vi "AutoFileCreatorMain.vi"() -> ()   [LabVIEW 2017]
uses:
  <vilib>/Utility/inputDevices.llb/mouseAcquire.vi
  <vilib>/xml/NI_XML.lvlib
  <resource>/objmgr/DOMUserDefRef.rc
panel:
  out "CopiedData":string
  in  "LocalFileNames":string[](array[string])=["1A.txt", "1B.txt", "1C.txt", "1D.txt", "2A.txt", "2B.txt", "2C.txt", "2D.txt", "3A.txt", "3B.txt", "3C.txt", "3D.txt", "4A.txt", "4B.txt", "4C.txt", "4D.txt"]
  out "standard output":string
  out "standard error":string="NI Linux Real-Time (run mode)\n\nLog in with your NI-Auth credentials.\n\n"
  in  "LocalFiles":i32(listbox)=2
  in  "SaveToLocal":bool
  in  "LoadFromLocal":bool
  in  "ExportToRobot":bool
  out "XML With IDs":string="<Sequential ID=\"1\">\n</Sequential>"
  in  "Commands":i32(listbox)=-1
  out "XML":string="<Sequential>\n</Sequential>"
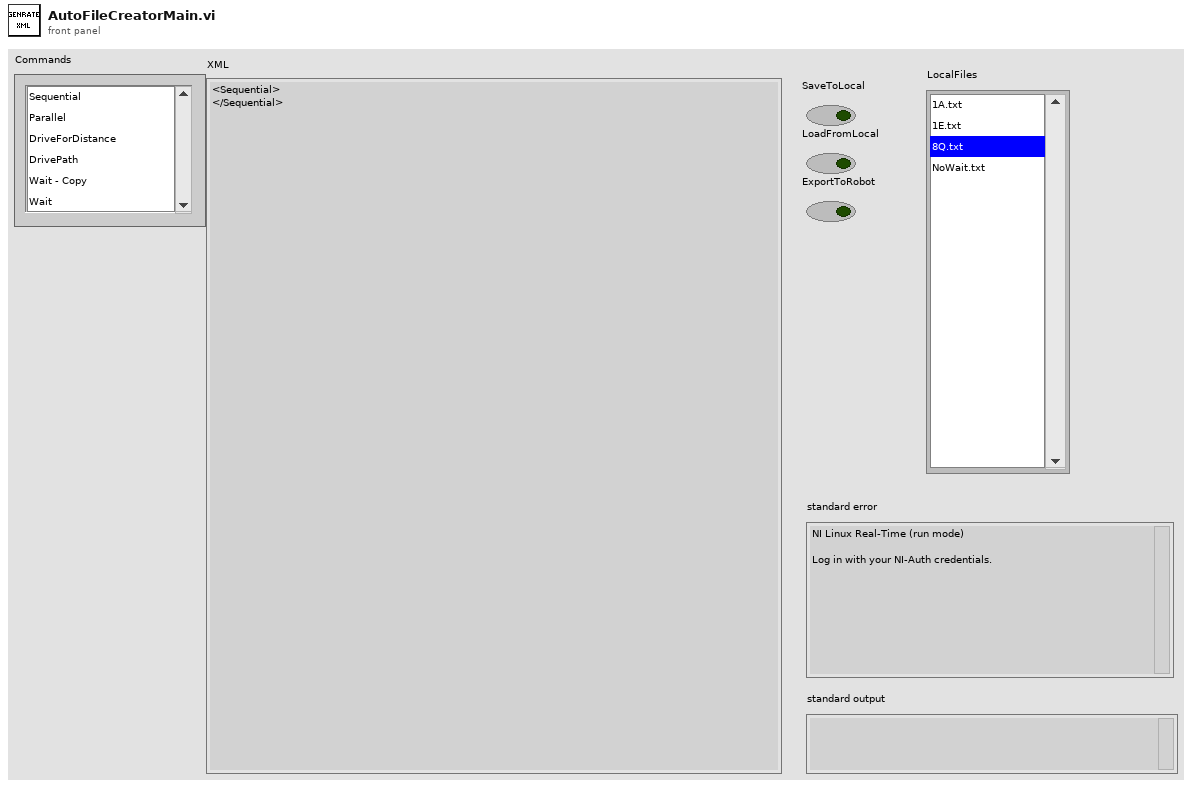
[diagram p1: front panel]
types:
  T1 = cluster{"Horizontal":i32, "Vertical":i32, "Scrolling":i32}
  T2 = typedef "eventvkey.ctl" = enum16{"ASCII", "Enter", "Return", "Shift", "Ctrl", "Alt", "Cmd", "Opt", "Caps", "NumLock", "Clear", "Break", "Up", "Down", "Left", "Right", "Insert", "Delete", "Home", "End", "PageUp", "PageDown", "Escape", "Help", "Pause", "ScrollLock", "F1", "F2", "F3", "F4", "F5", "F6", "F7", "F8", "F9", "F10", "F11", "F12", "F13", "F14", "F15", "F16", "F17", "F18", "F19", "F20", "F21", "F22", "F23", "F24", "Play", "VolumeUp", "VolumeDown", "Mute", "Two Byte Char"}
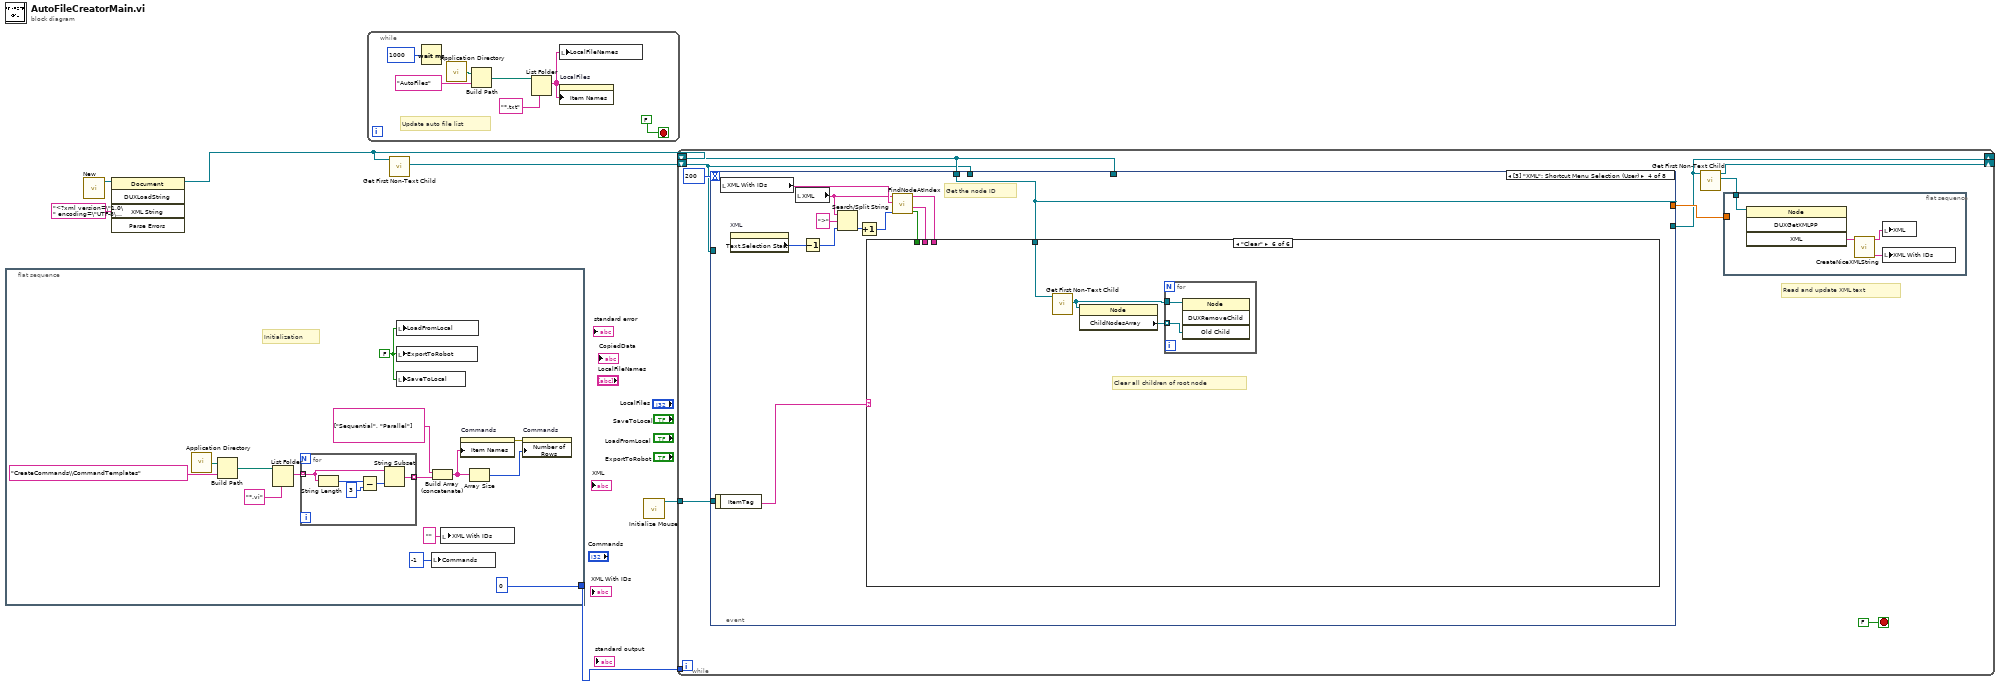
[diagram p0: block diagram]
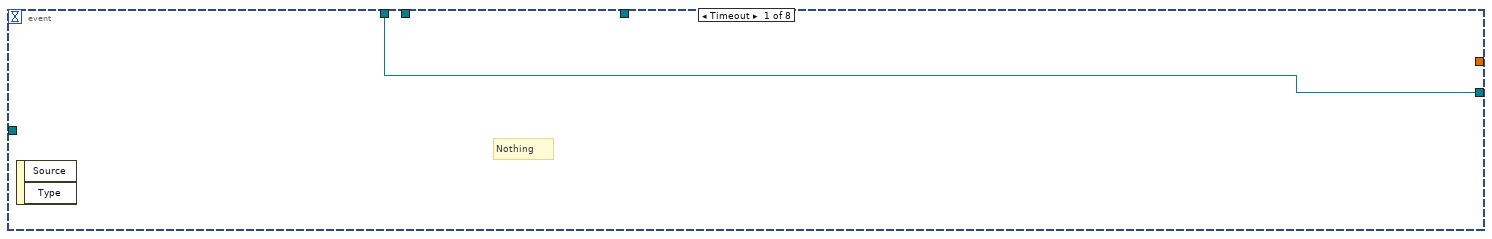
[diagram p2: hidden frame]
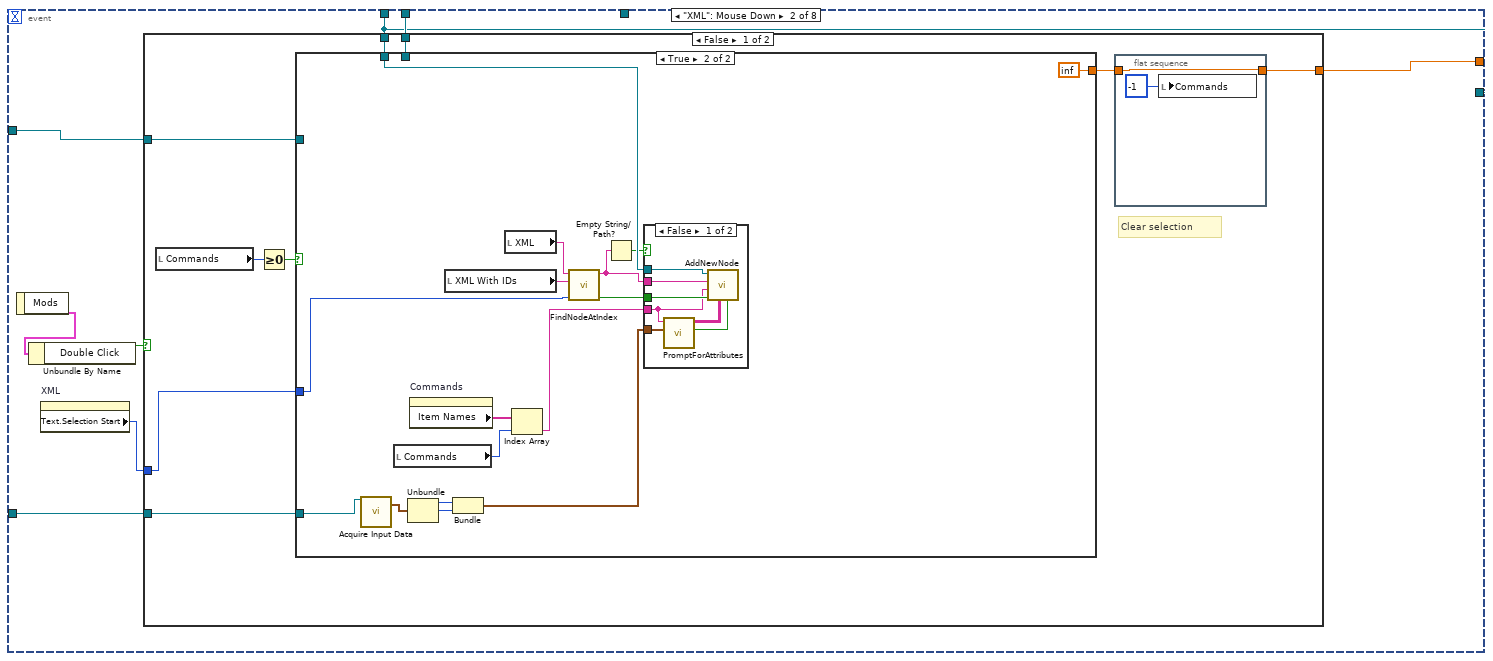
[diagram p3: hidden frame]
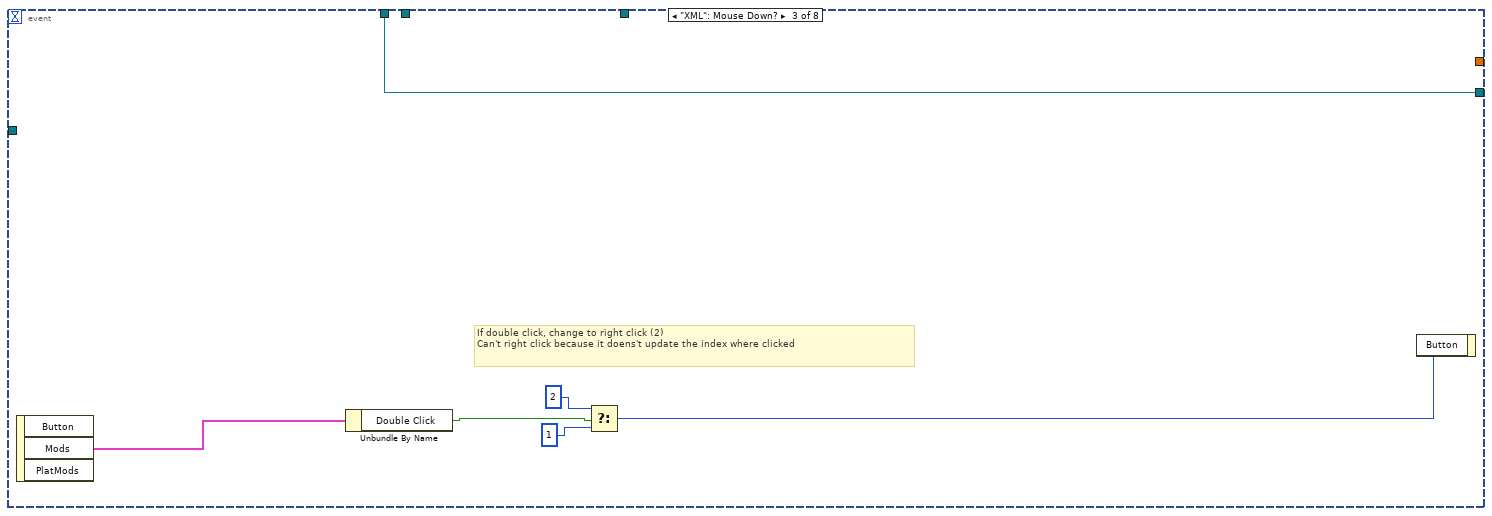
[diagram p7: hidden frame]
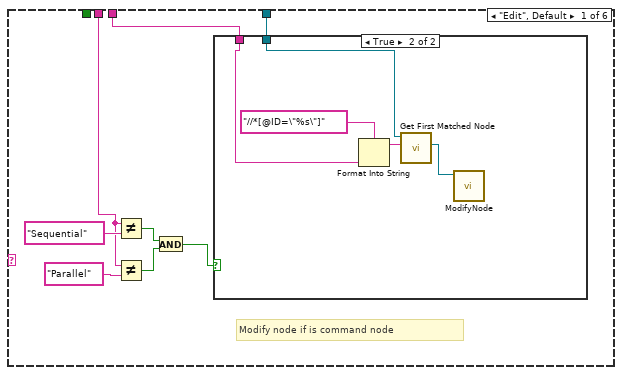
[diagram p8: hidden frame]
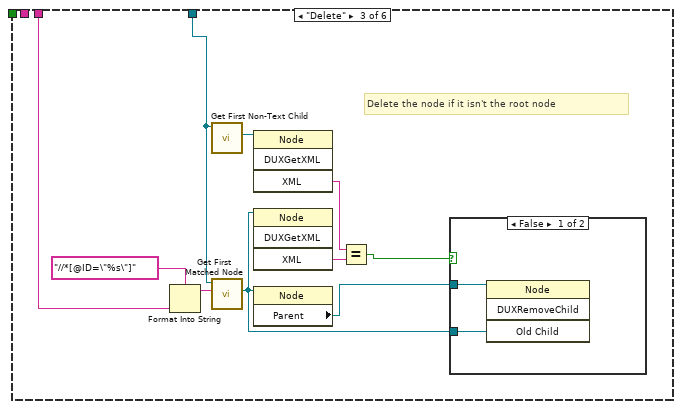
[diagram p11: hidden frame]
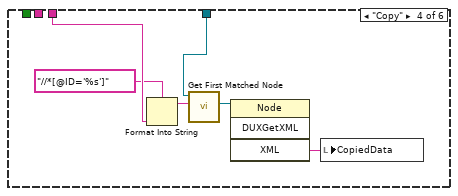
[diagram p13: hidden frame]
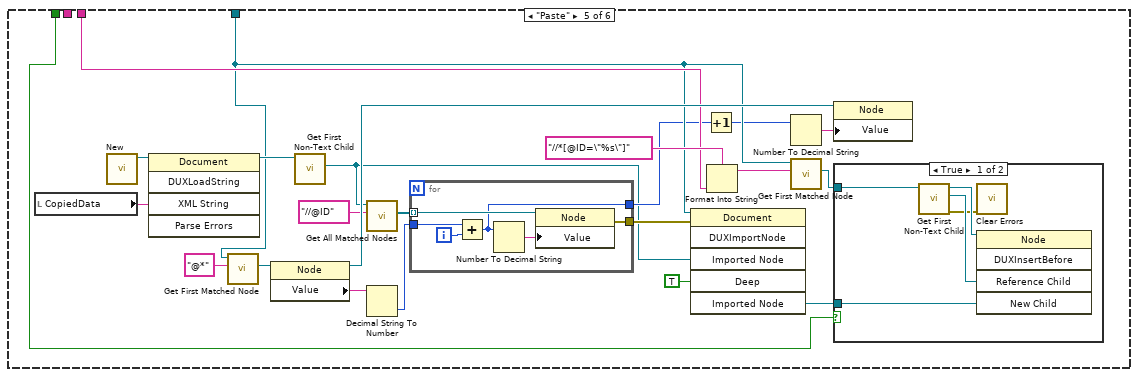
[diagram p14: hidden frame]
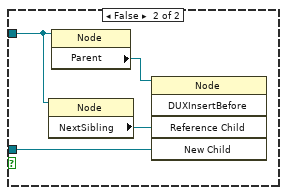
[diagram p15: hidden frame]
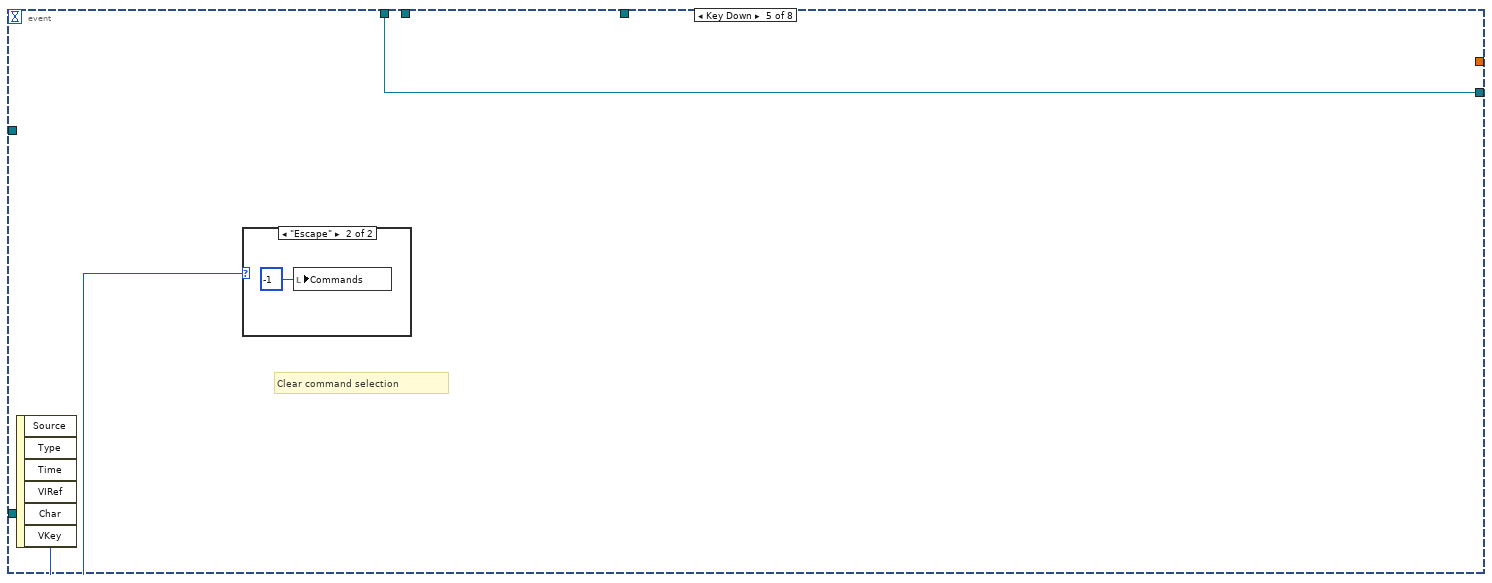
[diagram p16: hidden frame]
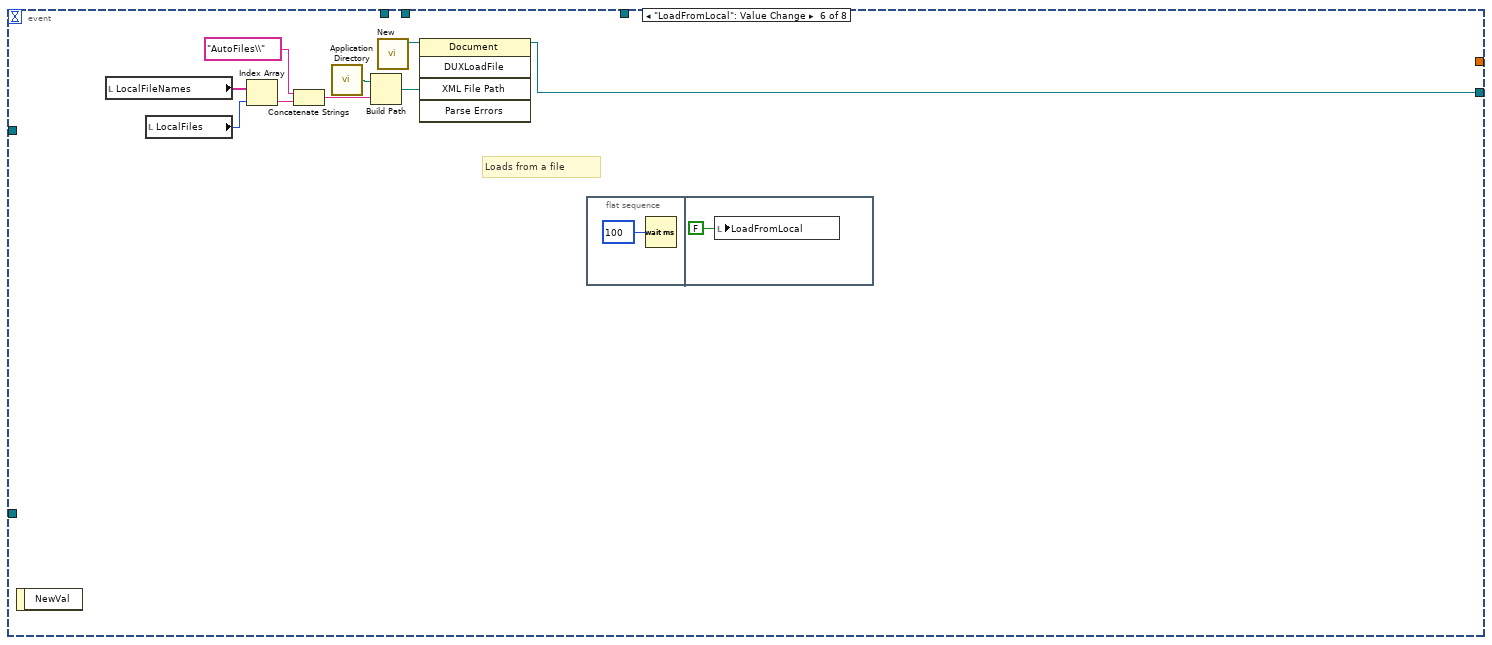
[diagram p18: hidden frame]
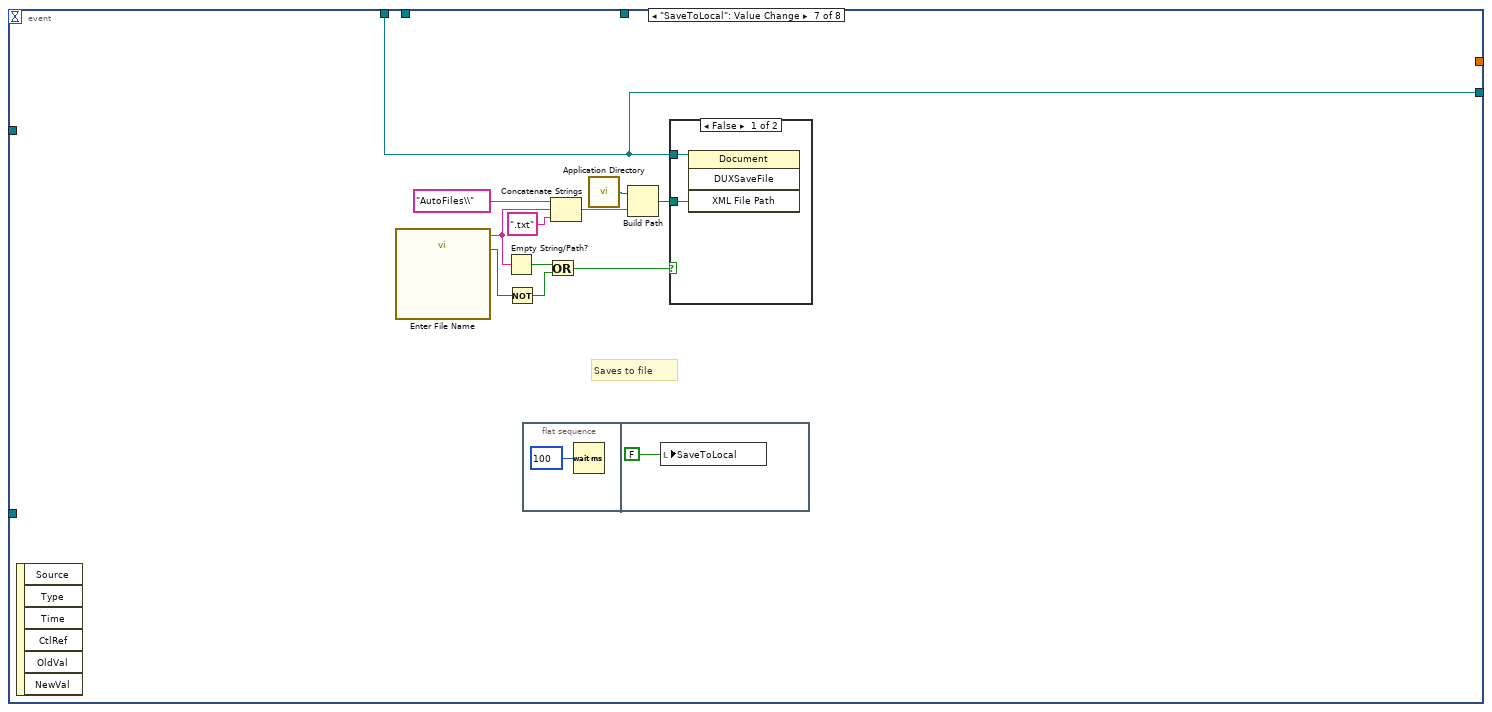
[diagram p19: hidden frame]
diagram:
  n1 = flat-sequence {
    tunnel: [0] -> w6
    frame #0 {
      w7 = FALSE ("SaveToLocal")
      # "Initialization"
      n2 = call <vilib>:"Application Directory.vi"() -> ("Application Directory"=w11:path)
      n3 = Build Path(base path=w11, name or relative path="CreateCommands\\CommandTemplates") -> (appended path=w12:path)
      n4 = List Folder(path=w12, pattern="*.vi") -> (filenames=w13:string[])  [unwired: 2 in, 3 out]
      n5 = for {
        tunnel: w13 -> [w25] mode=indexing
        tunnel: [w21] -> w14 mode=indexing
        n6 = String Length(string=w25) -> (length=w24:i32)
        n7 = Subtract(x=w24, y=3) -> (x-y=w22:i32)
        n8 = String Subset(string=w25, length (rest)=w22) -> (substring=w21:string)  [unwired: 1 in]
      }
      n9 = local write "LoadFromLocal"(w7) -> ()
      n10 = local write "ExportToRobot"(w7) -> ()
      n11 = local write "SaveToLocal"(w7) -> ()
      n12 = local write "Commands"(-1 ("Active Row:Active Row Number")) -> ()
      n13 = Build Array (concatenate)(string[] ["Sequential", "Parallel"], w14) -> (w15:string[])
      n14 = local write "XML With IDs"("" ("XML With IDs")) -> ()
      n15 = property on="Commands" class="LstBox (strict)"("Item Names"=w15) -> (error out=w17:errorcluster)  [unwired: 2 in, 1 out]
      n16 = Array Size(array=w15) -> (size(s)=w16:i32)
      n17 = property on="Commands" class="LstBox (strict)"(error in=w17, "Number of Rows"=w16) -> ()  [unwired: 1 in, 2 out]
    }
  }
  n18 = call <vilib>:"New.vi"() -> ("DOM document out"=w5:refnum<k20>)  [unwired: 8 in, 1 out]
  n19 = invoke class="Document" method="DUXLoadString"(reference=w5, "XML String"="<?xml version=\"1.0\" encoding=\"UTF-8\"?><Sequential ID=\"1\"></Sequential>") -> (reference out=w4:refnum<k20>)  [unwired: 3 in, 4 out]
  n20 = while {
    stop <- FALSE stop-if-true
    # "Update auto file list"
    n21 = Wait (ms)(milliseconds to wait=u32 1000) -> ()  [unwired: 1 out]
    n22 = call <vilib>:"Application Directory.vi"() -> ("Application Directory"=w27:path)
    n23 = Build Path(base path=w27, name or relative path="AutoFiles") -> (appended path=w32:path)
    n24 = List Folder(path=w32, pattern="*.txt") -> (filenames=w26:string[])  [unwired: 2 in, 3 out]
    n25 = local write "LocalFileNames"(w26) -> ()
    n26 = property on="LocalFiles" class="LstBox (strict)"("Item Names"=w26) -> ()  [unwired: 2 in, 2 out]
  }
  n27 = call <vilib>:"Get First Non-Text Child.vi"("node in"=w4) -> ("child node"=w3:refnum<k20>)  [unwired: 7 in, 3 out]
  n28 = call <vilib>:"Initialize Mouse.vi"() -> ("device ID"=w2:refnum<k1>)  [unwired: 10 in, 1 out]
  n29 = while {
    tunnel: w6 -> [_]
    shift-right: [w33] -> _
    shift-left: w4 -> [w37]
    shift-right: [w35] -> _
    shift-left: w3 -> [w36]
    tunnel: w2 -> [w38]
    stop <- FALSE stop-if-true
    # "Read and update XML text"
    n30 = event shown="[3] \"XML\": Shortcut Menu Selection (User)" {
      selector: _ -> [_ _ _ _ _ _ _ _]
      dyn-events: _ -> [_ _ _ _ _ _ _ _]
      timeout: 200 -> [_ _ _ _ _ _ _ _]
      tunnel: w36 -> [_ w54 _ _ _ _ _ _]
      tunnel: w37 -> [w46 w47 w89 w96 w181 _ w195 w210]
      tunnel: w36 -> [_ w53 _ _ _ _ _ _]
      tunnel: [_ w52 _ _ _ _ _ _] -> w39
      tunnel: w38 -> [_ w51 _ _ _ _ _ _]
      tunnel: w37 -> [_ _ _ _ _ _ _ _]
      tunnel: [w46 w47 w89 w96 w181 w184 w195 w210] -> w33
      event Timeout {
        # "Nothing"
        n31 = event-data() -> ()  [unwired: 1 in, 2 out]
      }
      event "XML": Mouse Down {
        n32 = event-data() -> ("Mods"=w50:cluster{"Double Click":bool, "Menu Key":bool})  [unwired: 1 in]
        n33 = Unbundle By Name(w50) -> ("Double Click"=w49:bool)
        n34 = property on="XML" class="Str"() -> ("Text.Selection Start"=w48:u32)  [unwired: 2 in, 2 out]
        n35 = case shown="False" w49 {
          tunnel: w54 -> [w61 _]
          tunnel: w47 -> [w60 _]
          tunnel: w53 -> [w59 _]
          tunnel: [w57 _] -> w52
          tunnel: w51 -> [w56 _]
          tunnel: w48 -> [w55 _]
          frame False {
            # "Clear selection"
            n36 = local read "Commands"() -> (w63:i32)
            n37 = Greater Or Equal To 0?(x=w63) -> (x >= 0?=w62:bool)
            n38 = case shown="True" w62 {
              tunnel: w61 -> [_ _]
              tunnel: w60 -> [_ w72]
              tunnel: w59 -> [_ _]
              tunnel: w55 -> [_ w76]
              tunnel: [_ inf] -> w58
              tunnel: w56 -> [_ w70]
              frame False {
              }
              frame True {
                n39 = call-poly <vilib>:"Acquire Input Data.vi"("device ID"=w70) -> ("axis info"=w69:T1)  [unwired: 15 in, 3 out]
                n40 = local read "Commands"() -> (w78:i32)
                n41 = Unbundle(w69) -> ("Horizontal"=w68:i32, "Vertical"=w67:i32)  [unwired: 1 out]
                n42 = property on="Commands" class="LstBox (strict)"() -> ("Item Names"=w79:string[])  [unwired: 2 in, 2 out]
                n43 = local read "XML With IDs"() -> (w75:string)
                n44 = Bundle("Horizontal"=w68, "Vertical"=w67) -> (w64:cluster{"Horizontal":i32, "Vertical":i32})  [unwired: 1 in]
                n45 = local read "XML"() -> (w74:string)
                n46 = Index Array(array=w79, index=w78) -> (element=w71:string)
                n47 = call "FindNodeAtIndex.vi"("ClickIndex"=w76, "XML with IDs"=w75, "XML In"=w74) -> ("Insert as child not sibling"=w73:bool, "Node ID"=w66:string)  [unwired: 6 in, 1 out]
                n48 = Empty String/Path?(string/path=w66) -> (empty?=w65:bool)
                n49 = case shown="False" w65 {
                  tunnel: w73 -> [w86 _]
                  tunnel: w72 -> [w85 _]
                  tunnel: w71 -> [w82 _]
                  tunnel: w66 -> [w84 _]
                  tunnel: w64 -> [w83 _]
                  frame False {
                    n50 = call "PromptForAttributes.vi"("Mouse Coords"=w83, "New Node Name"=w82) -> ("Canceled"=w81:bool, "Attributes"=w80:string[][])  [unwired: 8 in]
                    n51 = call "AddNewNode.vi"("Cancel"=w81, "Attributes"=w80, "Insert As Child"=w86, "New Node Name"=w82, "Node ID"=w84, "DOM document"=w85) -> ()  [unwired: 6 in]
                  }
                  frame True {
                  }
                }
              }
            }
            n52 = flat-sequence {
              tunnel: w58 -> [w87]
              tunnel: [w87] -> w57
              frame #0 {
                n53 = local write "Commands"(-1 ("Active Row:Active Row Number")) -> ()
              }
            }
          }
          frame True {
            # "Leave double clicking to that other event case"
          }
        }
      }
      event "XML": Mouse Down? {
        # "If double click, change to right click (2)\nCan't right click because it doens't update the index where clicked"
        n54 = event-data() -> ("Mods"=w94:cluster{"Double Click":bool, "Menu Key":bool})  [unwired: 1 in, 2 out]
        n55 = Unbundle By Name(w94) -> ("Double Click"=w93:bool)
        n56 = Select(t=u16 2 ("Button"), s=w93, f=u16 1 ("Button")) -> (s? t:f=w90:u16)
        n57 = event-data("Button"=w90) -> ()  [unwired: 1 in, 1 out]
      }
      event "XML": Shortcut Menu Selection (User) {
        # "Get the node ID"
        n58 = event-data() -> ("ItemTag"=w101:string)  [unwired: 1 in]
        n59 = local read "XML With IDs"() -> (w98:string)
        n60 = property on="XML" class="Str"() -> ("Text.Selection Start"=w106:u32)  [unwired: 2 in, 2 out]
        n61 = local read "XML"() -> (w97:string)
        n62 = Decrement(x=w106) -> (x-1=w104:u32)
        n63 = Search/Split String(string=w97, search string/char (-)=">", offset (0)=w104) -> (offset of match=w102:i32)  [unwired: 2 out]
        n64 = Increment(x=w102) -> (x+1=w103:i32)
        n65 = call "FindNodeAtIndex.vi"("ClickIndex"=w103, "XML with IDs"=w98, "XML In"=w97) -> ("Insert as child not sibling"=w95:bool, "Node Name"=w99:string, "Node ID"=w100:string)  [unwired: 6 in]
        n66 = case shown="\"Clear\"" w101 {
          tunnel: w100 -> [w114 _ w127 w136 w147 _]
          tunnel: w96 -> [w113 _ w120 w137 w146 w178]
          tunnel: w99 -> [w110 _ _ _ _ _]
          tunnel: w95 -> [_ _ _ _ w154 _]
          frame "Edit", Default {
            # "Modify node if is command node"
            n67 = Not Equal?(x=w110, y="Sequential") -> (x != y?=w111:bool)
            n68 = Not Equal?(x=w110, y="Parallel") -> (x != y?=w108:bool)
            n69 = And(x=w111, y=w108) -> (x .and. y?=w107:bool)
            n70 = case shown="True" w107 {
              tunnel: w114 -> [_ w117]
              tunnel: w113 -> [_ w115]
              frame False {
              }
              frame True {
                n71 = Format Into String(format string="//*[@ID=\"%s\"]", w117) -> (resulting string=w119:string)  [unwired: 2 in, 1 out]
                n72 = call <vilib>:"Get First Matched Node.vi"("XPath expression"=w119, "node in"=w115) -> ("node result"=w116:refnum<k20>)  [unwired: 7 in, 2 out]
                n73 = call "ModifyNode.vi"("Node"=w116) -> ()  [unwired: 11 in]
              }
            }
          }
          frame "Move" {
            # "Not implemented yet"
          }
          frame "Delete" {
            # "Delete the node if it isn't the root node"
            n74 = Format Into String(format string="//*[@ID=\"%s\"]", w127) -> (resulting string=w129:string)  [unwired: 2 in, 1 out]
            n75 = call <vilib>:"Get First Non-Text Child.vi"("node in"=w120) -> ("child node"=w125:refnum<k20>)  [unwired: 7 in, 3 out]
            n76 = call <vilib>:"Get First Matched Node.vi"("XPath expression"=w129, "node in"=w120) -> ("node result"=w123:refnum<k20>)  [unwired: 7 in, 2 out]
            n77 = invoke class="Node" method="DUXGetXML"(reference=w125) -> ("XML"=w124:string)  [unwired: 3 in, 3 out]
            n78 = invoke class="Node" method="DUXGetXML"(reference=w123) -> ("XML"=w122:string)  [unwired: 3 in, 3 out]
            n79 = property class="Node"(reference=w123) -> ("Parent"=w126:refnum<k20>)  [unwired: 1 in, 2 out]
            n80 = Equal?(x=w124, y=w122) -> (x = y?=w121:bool)
            n81 = case shown="False" w121 {
              tunnel: w126 -> [w131 _]
              tunnel: w123 -> [w130 _]
              frame False {
                n82 = invoke class="Node" method="DUXRemoveChild"(reference=w131, "Old Child"=w130) -> ()  [unwired: 2 in, 4 out]
              }
              frame True {
              }
            }
          }
          frame "Copy" {
            n83 = Format Into String(format string="//*[@ID='%s']", w136) -> (resulting string=w134:string)  [unwired: 2 in, 1 out]
            n84 = call <vilib>:"Get First Matched Node.vi"("XPath expression"=w134, "node in"=w137) -> ("node result"=w133:refnum<k20>)  [unwired: 7 in, 2 out]
            n85 = invoke class="Node" method="DUXGetXML"(reference=w133) -> ("XML"=w132:string)  [unwired: 3 in, 3 out]
            n86 = local write "CopiedData"(w132) -> ()
          }
          frame "Paste" {
            n87 = local read "CopiedData"() -> (w159:string)
            n88 = call <vilib>:"New.vi"() -> ("DOM document out"=w160:refnum<k20>)  [unwired: 8 in, 1 out]
            n89 = invoke class="Document" method="DUXLoadString"(reference=w160, "XML String"=w159) -> (reference out=w158:refnum<k20>)  [unwired: 3 in, 4 out]
            n90 = call <vilib>:"Get First Matched Node.vi"("XPath expression"="@*", "node in"=w146) -> ("node result"=w152:refnum<k20>)  [unwired: 7 in, 2 out]
            n91 = property class="Node"(reference=w152) -> (reference out=w148:refnum<k20>, "Value"=w150:string)  [unwired: 1 in, 1 out]
            n92 = call <vilib>:"Get First Non-Text Child.vi"("node in"=w158) -> ("child node"=w138:refnum<k20>)  [unwired: 7 in, 3 out]
            n93 = call <vilib>:"Get All Matched Nodes.vi"("XPath expression"="//@ID", "node in"=w138) -> ("node result array"=w143:refnum<k20>[])  [unwired: 7 in, 2 out]
            n94 = Decimal String To Number(string=w150) -> (number=w140:i32)  [unwired: 2 in, 1 out]
            n95 = for {
              tunnel: w143 -> [w166] mode=indexing
              tunnel: [w164] -> w142
              tunnel: w140 -> [w162]
              tunnel: [w161] -> w139
              i -> [w165]
              n96 = Add(x=w162, y=w165) -> (x+y=w164:i32)
              n97 = Number To Decimal String(number=w164) -> (decimal integer string=w163:string)  [unwired: 1 in]
              n98 = property class="Node"(reference=w166, "Value"=w163) -> (error out=w161:errorcluster)  [unwired: 1 in, 1 out]
            }
            n99 = invoke class="Document" method="DUXImportNode"(reference=w146, error in=w139, "Imported Node"=w138, "Deep"=TRUE) -> ("Imported Node"=w145:refnum<k20>)  [unwired: 2 in, 5 out]
            n100 = Increment(x=w142) -> (x+1=w141:i32)
            n101 = Format Into String(format string="//*[@ID=\"%s\"]", w147) -> (resulting string=w156:string)  [unwired: 2 in, 1 out]
            n102 = Number To Decimal String(number=w141) -> (decimal integer string=w149:string)  [unwired: 1 in]
            n103 = call <vilib>:"Get First Matched Node.vi"("XPath expression"=w156, "node in"=w146) -> ("node result"=w155:refnum<k20>)  [unwired: 7 in, 2 out]
            n104 = property class="Node"(reference=w148, "Value"=w149) -> ()  [unwired: 1 in, 2 out]
            n105 = case shown="True" w154 {
              tunnel: w155 -> [w168 w174]
              tunnel: w145 -> [w167 w172]
              frame True {
                n106 = call <vilib>:"Get First Non-Text Child.vi"("node in"=w168) -> ("error out"=w169:errorcluster, "child node"=w170:refnum<k20>, "node out"=w171:refnum<k20>)  [unwired: 7 in, 1 out]
                n107 = call <vilib>:"Clear Errors.vi"("error in (no error)"=w169) -> ()  [unwired: 5 in, 2 out]
                n108 = invoke class="Node" method="DUXInsertBefore"(reference=w171, "Reference Child"=w170, "New Child"=w167) -> ()  [unwired: 2 in, 5 out]
              }
              frame False {
                n109 = property class="Node"(reference=w174) -> ("NextSibling"=w175:refnum<k20>)  [unwired: 1 in, 2 out]
                n110 = property class="Node"(reference=w174) -> ("Parent"=w173:refnum<k20>)  [unwired: 1 in, 2 out]
                n111 = invoke class="Node" method="DUXInsertBefore"(reference=w173, "Reference Child"=w175, "New Child"=w172) -> ()  [unwired: 2 in, 5 out]
              }
            }
          }
          frame "Clear" {
            # "Clear all children of root node"
            n112 = call <vilib>:"Get First Non-Text Child.vi"("node in"=w178) -> ("child node"=w176:refnum<k20>)  [unwired: 7 in, 3 out]
            n113 = property class="Node"(reference=w176) -> ("ChildNodesArray"=w177:refnum<k20>[])  [unwired: 1 in, 2 out]
            n114 = for {
              tunnel: w176 -> [w180]
              tunnel: w177 -> [w179] mode=indexing
              n115 = invoke class="Node" method="DUXRemoveChild"(reference=w180, "Old Child"=w179) -> ()  [unwired: 2 in, 4 out]
            }
          }
        }
      }
      event Key Down {
        # "Clear command selection"
        n116 = event-data() -> ("VKey"=w182:T2)  [unwired: 1 in, 5 out]
        n117 = case shown="\"Escape\"" w182 {
          frame "ASCII", Default {
          }
          frame "Escape" {
            n118 = local write "Commands"(-1 ("Active Row:Active Row Number")) -> ()
          }
        }
      }
      event "LoadFromLocal": Value Change {
        # "Loads from a file"
        n119 = event-data() -> ()  [unwired: 1 in, 1 out]
        n120 = local read "LocalFileNames"() -> (w192:string[])
        n121 = local read "LocalFiles"() -> (w191:i32)
        n122 = Index Array(array=w192, index=w191) -> (element=w187:string)
        n123 = Concatenate Strings("AutoFiles\\" ("string"), w187) -> (w185:string)
        n124 = call <vilib>:"Application Directory.vi"() -> ("Application Directory"=w190:path)
        n125 = Build Path(base path=w190, name or relative path=w185) -> (appended path=w189:path)
        n126 = call <vilib>:"New.vi"() -> ("DOM document out"=w188:refnum<k20>)  [unwired: 8 in, 1 out]
        n127 = invoke class="Document" method="DUXLoadFile"(reference=w188, "XML File Path"=w189) -> (reference out=w184:refnum<k20>)  [unwired: 3 in, 4 out]
        n128 = flat-sequence {
          frame #0 {
            n129 = Wait (ms)(milliseconds to wait=u32 100) -> ()  [unwired: 1 out]
          }
          frame #1 {
            n130 = local write "LoadFromLocal"(FALSE ("SaveToLocal")) -> ()
          }
        }
      }
      event "SaveToLocal": Value Change {
        # "Saves to file"
        n131 = event-data() -> ()  [unwired: 1 in, 6 out]
        n132 = call "Enter File Name"() -> ("File Name"=w197:string, "Enter"=w203:bool)  [unwired: 17 in, 1 out]
        n133 = Empty String/Path?(string/path=w197) -> (empty?=w205:bool)
        n134 = Not(x=w203) -> (.not. x?=w204:bool)
        n135 = flat-sequence {
          frame #0 {
            n136 = Wait (ms)(milliseconds to wait=u32 100) -> ()  [unwired: 1 out]
          }
          frame #1 {
            n137 = local write "SaveToLocal"(FALSE ("SaveToLocal")) -> ()
          }
        }
        n138 = Or(x=w205, y=w204) -> (x .or. y?=w196:bool)
        n139 = Concatenate Strings("AutoFiles\\" ("name or relative path"), w197, ".txt" ("string")) -> (w200:string)
        n140 = call <vilib>:"Application Directory.vi"() -> ("Application Directory"=w199:path)
        n141 = Build Path(base path=w199, name or relative path=w200) -> (appended path=w198:path)
        n142 = case shown="False" w196 {
          tunnel: w195 -> [w207 _]
          tunnel: w198 -> [w206 _]
          frame False {
            n143 = invoke class="Document" method="DUXSaveFile"(reference=w207, "XML File Path"=w206) -> ()  [unwired: 2 in, 4 out]
          }
          frame True {
          }
        }
      }
      event "ExportToRobot": Value Change {
        # "Exports to robot"
        # "replace backslash with slash\nand change begining to /c/"
        n144 = event-data() -> ()  [unwired: 1 in, 6 out]
        n145 = local read "LocalFileNames"() -> (w230:string[])
        n146 = local read "LocalFiles"() -> (w229:i32)
        n147 = Index Array(array=w230, index=w229) -> (element=w231:string)
        n148 = Build Path(name or relative path="AutoFiles") -> (appended path=w232:path)  [unwired: 1 in]
        n149 = Build Path(base path=w232, name or relative path=w231) -> (appended path=w213:path)
        n150 = Path To String(path=w213) -> (string=w220:string)
        n151 = String Subset(string=w220, offset (0)=2) -> (substring=w218:string)  [unwired: 1 in]
        n152 = Search and Replace String(replace all?=TRUE ("replace all? (F)"), input string=w218, search string="\\", replace string="/" ("replace string (\"\")")) -> (result string=w217:string)  [unwired: 4 in, 3 out]
        n153 = Concatenate Strings("\"/c" ("string"), w217, "\"" ("string")) -> (w215:string)
        n154 = Concatenate Strings("\"C:\\Program Files\\Git\\usr\\bin\\scp.exe\" " ("command line"), w215, " lvuser@roboRIO-1712-FRC.local:/home/lvuser/Auto/AutoFiles" ("string")) -> (w224:string)
        n155 = call <vilib>:"System Exec.vi"("wait until completion? (T)"=TRUE, "command line"=w224) -> ("standard error"=w211:string, "standard output"=w212:string)  [unwired: 6 in, 2 out]
        n156 = local write "standard error"(w211) -> ()
        n157 = local write "standard output"(w212) -> ()
        n158 = flat-sequence {
          tunnel: w211 -> [_]
          frame #0 {
            n159 = local write "ExportToRobot"(FALSE ("ExportToRobot")) -> ()
          }
        }
      }
    }
    n160 = call <vilib>:"Get First Non-Text Child.vi"("node in"=w33) -> ("child node"=w34:refnum<k20>, "node out"=w35:refnum<k20>)  [unwired: 7 in, 2 out]
    n161 = flat-sequence {
      tunnel: w39 -> [_]
      tunnel: w34 -> [w42]
      frame #0 {
        n162 = invoke class="Node" method="DUXGetXMLPP"(reference=w42) -> ("XML"=w43:string)  [unwired: 3 in, 3 out]
        n163 = call "CreateNiceXMLString.vi"("XML In"=w43) -> ("XML String With IDs"=w44:string, "XML String Human Readable"=w45:string)  [unwired: 9 in]
        n164 = local write "XML"(w45) -> ()
        n165 = local write "XML With IDs"(w44) -> ()
      }
    }
  }
